vi "rqcAlice SPI.Set Att Value.vi"(8 "error in":errorcluster, 10 "Attenuation, dB":dbl, 11 "Alice FPGA Reference In":refnum<k20>) -> (0 "error out":errorcluster, 3 "Alice FPGA Reference Out":refnum<k20>)   [LabVIEW 2019]
uses:
  Shared/Shared Host Lib/SPI/typedefs/SPI.SubSystem.ctl
  <vilib>/Utility/error.llb/Error Cluster From Error Code.vi
  <vilib>/rvi/errors/niLvFpgaAdjustHostInterfaceError.vi
  <vilib>/rvi/interface/nirviReadWriteControl/nirviReadWriteControl.xnode
  NiFpgaLv.dll
  <vilib>/rvi/interface/Simulation/niFpgaSimulationCallBeginRW.vi
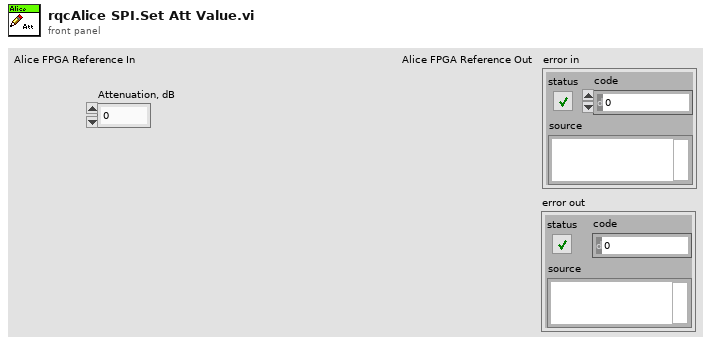
[diagram p1: front panel]
types:
  T1 = typedef "SPI.SubSystem.ctl" = enum8{"N/A", "DelayLine.MSB", "DelayLine.LSB", "Attenuation.dB", "Attenuation.DAC value", "SyncDetector.Offset", "SyncDetector.Comparator", "PM.Value[0]", "PM.Value[1]", "PM.Value[2]", "PM.Value[3]"}
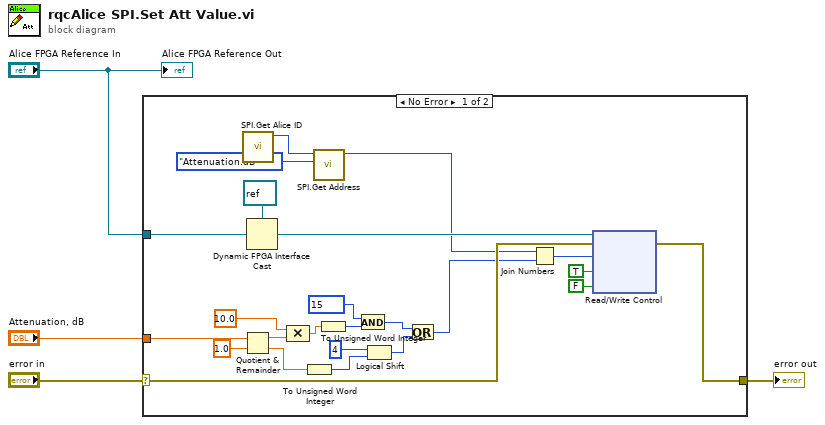
[diagram p0: block diagram]
diagram:
  n1 = case shown="No Error" "error in" {
    selector: "error in" -> [w22 w29]
    tunnel: [w18 w29] -> w3
    tunnel: "Alice FPGA Reference In" -> [w28 _]
    tunnel: "Attenuation, dB" -> [w17 _]
    frame No Error {
      n2 = call "SPI.Get Alice ID.vi"() -> ("Alice.ID"=w21:u8)  [unwired: 11 in]
      n3 = Quotient & Remainder(x=w17, y=1.0) -> (x-y*floor(x/y)=w15:dbl, floor(x/y)=w10:dbl)
      n4 = Dynamic FPGA Interface Cast(Session In=refnum<k20> refnum ("Type"), Type=w28) -> (Session Out=w23:refnum<k20>)
      n5 = Compound Arithmetic op=MULTIPLY(10.0 ("value"), w15) -> (w13:dbl)
      n6 = To Unsigned Word Integer(number=w10) -> (unsigned 16bit integer=w9:u16)
      n7 = call "SPI.Get Address.vi"("SPI.subSystem"=SPI.SubSystem."Attenuation.dB", "ID"=w21) -> ("Address"=w20:u16)  [unwired: 9 in]
      n8 = To Unsigned Word Integer(number=w13) -> (unsigned 16bit integer=w11:u16)
      n9 = And(x=u16 15, y=w11) -> (x .and. y?=w7:u16)
      n10 = Logical Shift(y=u16 4 ("x"), x=w9) -> (x << y=w6:u16)
      n11 = Or(x=w7, y=w6) -> (x .or. y?=w5:u16)
      n12 = Join Numbers(hi=w20, lo=w5) -> ((hi.lo)=w24:u32)
      n13 = xnode "Read/Write Control"("FPGA VI Reference In"=w23, "error in"=w22, "SPI.data"=w24, "SPI.write"=TRUE ("reset"), "SPI.write"=FALSE ("reset")) -> ("error out"=w18:errorcluster)  [unwired: 1 out]
    }
    frame Error {
    }
  }
  "error out" <- w3
  "Alice FPGA Reference Out" <- "Alice FPGA Reference In"
